vi "extract_noise.vi"(9 "Config":T2={"IO params"={"Conversion"={"Rate"=4.0, "In cards"=2, "Out channels"=4}, "Carriers"={"Phase shift"=180.0, "Levels"=[[0.8, 0.8, 0.8], [0.03, 0.03, 0.03]], "Delay samples"=73.15}}, "High rate STFT"={"Win param"=101.5, "Window type"=61, "Win order"=2, "DFT size"=64, "Channels"=[7], "Oversample"=64}, "Low rate STFT"={"Win param"=120.0, "Window type"=61, "Win order"=8, "DFT size"=64, "Channels"=[7], "Oversample"=64}, "Filtering"={"Hum"={"Frequency"=101.5, "Tc"=101.5, "Limit"=101.5, "FFT filter"=FALSE, "Detrend mode"=enum."Robust linear", "Enable"=FALSE}, "Kalman"={"Process noise"=101.5, "Measure noise"=101.5}, "Distortion"={"LF cut"=0.0, "Tc"=0.0, "Limit"=101.5, "FFT filter"=FALSE, "Detrend mode"=enum."Robust linear", "Enable"=FALSE}}} {"Filtering"."Distortion"."Limit" format="%#_3p"; "Filtering"."Distortion"."LF cut" format="%#_3p"; "Filtering"."Kalman"."Measure noise" format="%#_3p"; "Filtering"."Kalman"."Process noise" format="%#_3p"; "Filtering"."Hum"."Limit" format="%#_3p"; "Filtering"."Hum"."Frequency" format="%#_4p"; "Low rate STFT"."Oversample" min=1 step=1; "Low rate STFT"."Channels" min=0 step=1; "Low rate STFT"."DFT size" min=1 step=1; "Low rate STFT"."Window type" items=["Rectangle"=0, "Hanning"=1, "Hamming"=2, "Blackman-Harris"=3, "Exact Blackman"=4, "Blackman"=5, "Flat Top"=6, "4 Term B-Harris "=7, "7 Term B-Harris"=8, "Low Sidelobe"=9, "Blackman Nuttall"=11, "Triangle"=30, "Bartlett-Hanning"=31, "Bohman"=32, "Parzen"=33, "Welch"=34, "Kaiser"=60, "Dolph-Chebyshev"=61, "Gaussian"=62]; "High rate STFT"."Oversample" min=1 step=1; "High rate STFT"."Channels" min=0 step=1; "High rate STFT"."DFT size" min=1 step=1; "High rate STFT"."Window type" items=["Rectangle"=0, "Hanning"=1, "Hamming"=2, "Blackman-Harris"=3, "Exact Blackman"=4, "Blackman"=5, "Flat Top"=6, "4 Term B-Harris "=7, "7 Term B-Harris"=8, "Low Sidelobe"=9, "Blackman Nuttall"=11, "Triangle"=30, "Bartlett-Hanning"=31, "Bohman"=32, "Parzen"=33, "Welch"=34, "Kaiser"=60, "Dolph-Chebyshev"=61, "Gaussian"=62]; "IO params"."Carriers"."Levels" min=0.0 step=0.1; "IO params"."Conversion"."Rate" format="%#_8g"}, 10 "Modulation info":T1={"Fs full"=0.0, "Fs high"=0.0, "Fs low"=0.0, "Read size"=0, "FFT size low"=5000, "df low"=5000.0, "High carriers"=[], "Low carriers"=[], "Hi channels at low"=[7]} {"Hi channels at low" min=0 step=1; "Low carriers" format="%#_6p"; "High carriers" format="%#_6p"}, 11 "Spectrum":waveform(dbl)[](array[waveform])) -> (3 "Noise floor":dbl[][](array[numeric]) format="%#_6p")   [LabVIEW 2014]
uses:
  ilemt_config.ctl
  IO_params.ctl
  stft_params.ctl
  <vilib>/Analysis/4window.llb/windowTd.ctl
  filter_params.ctl
  detrend_mode.ctl
  modulation_info.ctl
  <vilib>/Analysis/NI_AALPro.lvlib
panel:
  out "Size (half FFT)":i32
  out "Waveform Graph":dbl[](graph)
  # "Find the noise floor on the spectrum display, defined as the median level within the band (high or low).  Does not do anything useful when displaying demodulated data."
  # "High"
  # "Low"
  # "X"
  # "Y"
  # "Z"
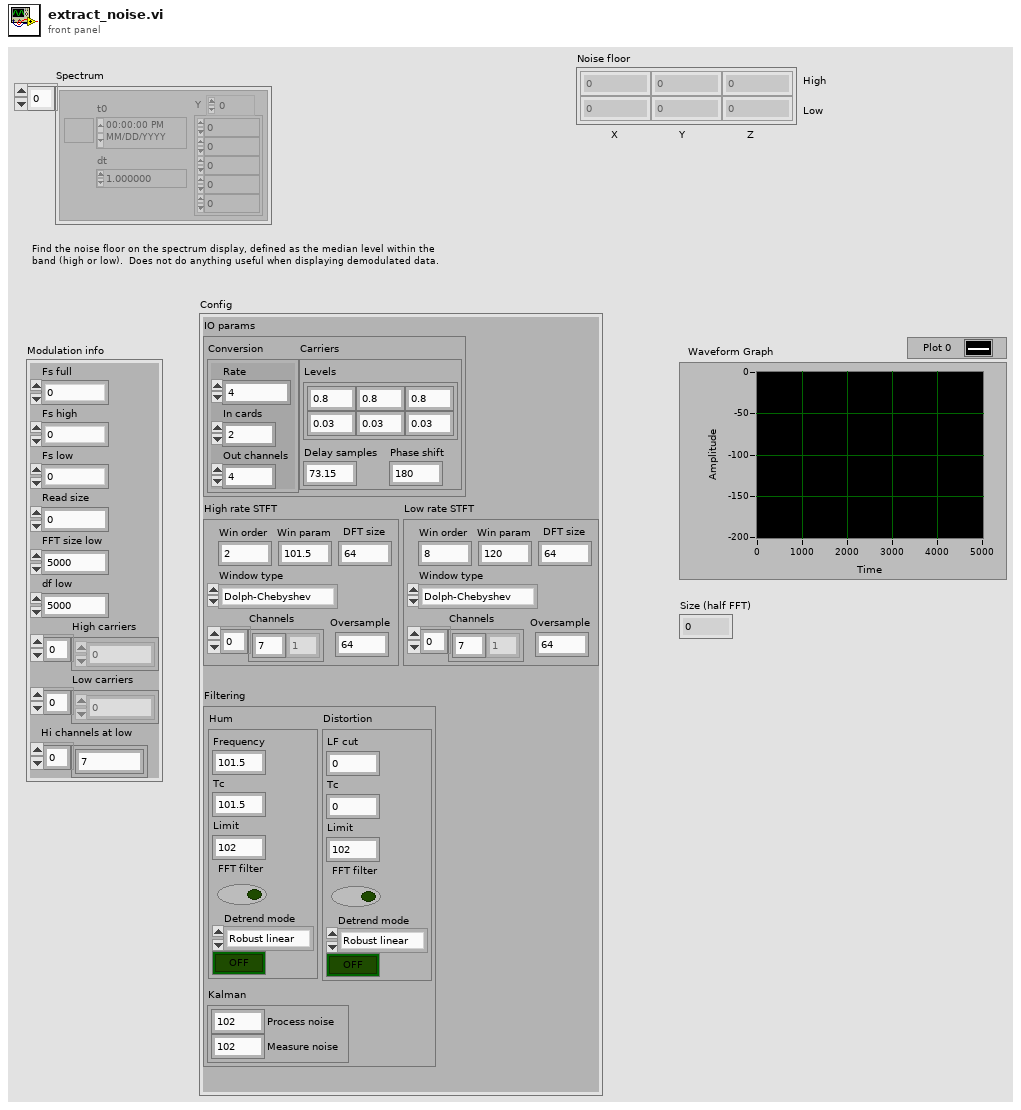
[diagram p1: front panel]
types:
  T1 = typedef "modulation_info.ctl" = cluster{"Fs full":dbl, "Fs high":dbl, "Fs low":dbl, "Read size":i32, "FFT size low":i32, "df low":dbl, "High carriers":dbl[], "Low carriers":dbl[], "Hi channels at low":i32[]}
  T2 = typedef "ilemt_config.ctl" = cluster{"IO params":T3, "High rate STFT":T4, "Low rate STFT":T4, "Filtering":T6}
  T3 = typedef "IO_params.ctl" = cluster{"Conversion":cluster{"Rate":dbl, "In cards":u32, "Out channels":u32}, "Carriers":cluster{"Phase shift":dbl, "Levels":dbl[][], "Delay samples":dbl}}
  T4 = typedef "stft_params.ctl" = cluster{"Win param":dbl, "Window type":T5, "Win order":i32, "DFT size":i32, "Channels":i32[], "Oversample":i32}
  T5 = typedef "NI_AALPro.lvlib/windowTd.ctl" = u32
  T6 = typedef "filter_params.ctl" = cluster{"Hum":cluster{"Frequency":dbl, "Tc":dbl, "Limit":dbl, "FFT filter":bool, "Detrend mode":T7, "Enable":bool}, "Kalman":cluster{"Process noise":dbl, "Measure noise":dbl}, "Distortion":cluster{"LF cut":dbl, "Tc":dbl, "Limit":dbl, "FFT filter":bool, "Detrend mode":T7, "Enable":bool}}
  T7 = typedef "detrend_mode.ctl" = enum16{"Zero mean", "Linear", "Robust linear"}
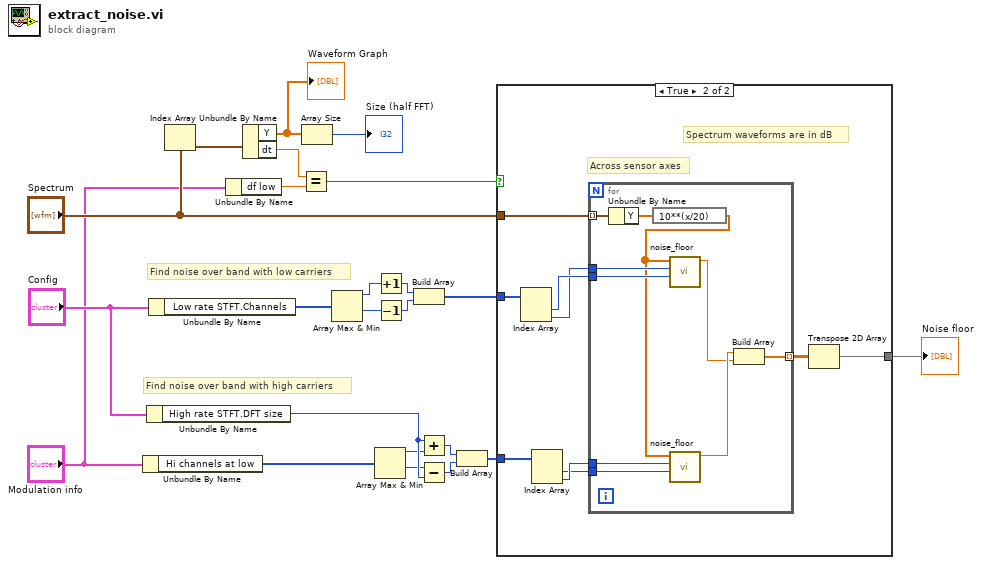
[diagram p0: block diagram]
diagram:
  # "Find noise over band with low carriers"
  # "Find noise over band with high carriers"
  n1 = Unbundle By Name("Modulation info") -> ("Hi channels at low"=w9:i32[])
  n2 = Unbundle By Name("Config") -> ("High rate STFT.DFT size"=w21:i32)
  n3 = Unbundle By Name("Config") -> ("Low rate STFT.Channels"=w23:i32[])
  n4 = Index Array(array="Spectrum") -> (element=w7:waveform(dbl))  [unwired: 1 in]
  n5 = Unbundle By Name("Modulation info") -> ("df low"=w3:dbl)
  n6 = Unbundle By Name(w7) -> ("Y"=w5:dbl[], "dt"=w2:dbl)
  "Waveform Graph" <- w5
  n7 = Equal?(x=w2, y=w3) -> (x = y?=w1:bool)
  n8 = Array Size(array=w5) -> (size(s)=→"Size (half FFT)":i32)
  n9 = Array Max & Min(array=w23) -> (max value=w16:i32, min value=w15:i32)  [unwired: 2 out]
  n10 = Array Max & Min(array=w9) -> (max value=w17:i32, min value=w18:i32)  [unwired: 2 out]
  n11 = Increment(x=w16) -> (x+1=w13:i32)
  n12 = Decrement(x=w15) -> (x-1=w14:i32)
  n13 = Build Array(w13, w14) -> (w12:i32[])
  n14 = Add(x=w21, y=w17) -> (x+y=w20:i32)
  n15 = Subtract(x=w18, y=w21) -> (x-y=w19:i32)
  n16 = Build Array(w20, w19) -> (w22:i32[])
  n17 = case shown="True" w1 {
    tunnel: w22 -> [_ w30]
    tunnel: w12 -> [_ w29]
    tunnel: [_ w25] -> w10
    tunnel: "Spectrum" -> [_ w24]
    frame False {
    }
    frame True {
      # "Across sensor axes"
      # "Spectrum waveforms are in dB"
      n18 = Index Array(array=w29) -> (element #1=w32:i32, element #2=w31:i32)  [unwired: 2 in]
      n19 = Index Array(array=w30) -> (element #1=w27:i32, element #2=w28:i32)  [unwired: 2 in]
      n20 = for {
        tunnel: w24 -> [w40] mode=indexing
        tunnel: w32 -> [w42]
        tunnel: w31 -> [w41]
        tunnel: w28 -> [w38]
        tunnel: w27 -> [w37]
        tunnel: [w33] -> w26 mode=indexing
        n21 = Unbundle By Name(w40) -> ("Y"=w39:dbl[])
        n22 = expression code="10**(x/20)"(w39) -> (w36:dbl[])
        n23 = call "noise_floor.vi"("Last bin"=w42, "First bin"=w41, "FFT"=w36) -> ("Noise floor"=w34:dbl)  [unwired: 8 in]
        n24 = call "noise_floor.vi"("Last bin"=w37, "First bin"=w38, "FFT"=w36) -> ("Noise floor"=w35:dbl)  [unwired: 8 in]
        n25 = Build Array(w35, w34) -> (w33:dbl[])
      }
      n26 = Transpose 2D Array(2D array=w26) -> (transposed array=w25:dbl[][])
    }
  }
  "Noise floor" <- w10
